vi "Set Dev Para wrapper.vi"(6 "iCurr":i32, 7 "iACR":i32, 8 "error in (no error)":errorcluster caption="错误输入（无错误）", 9 "iMCS":i32, 10 "dwCanNodeId":u32, 11 "dwDevIndex":u32) -> (0 "error out":errorcluster caption="错误输出", 3 "function return":u32)   [LabVIEW 2016, in "UISimCanFunc_wrapper.lvlib"]
doc: "_declspec (dllexport) DWORD SetDevPara_wrapper(DWORD dwDevIndex, DWORD dwCanNodeId, INT iMCS, INT iACR, INT iCurr);"
uses:
  <userlib>/UISimCanFunc_wrapper/UISimCanFunc_wrapper.lvlib
  <userlib>/UISimCanFunc_wrapper/UISimCanFunc_wrapper.dll
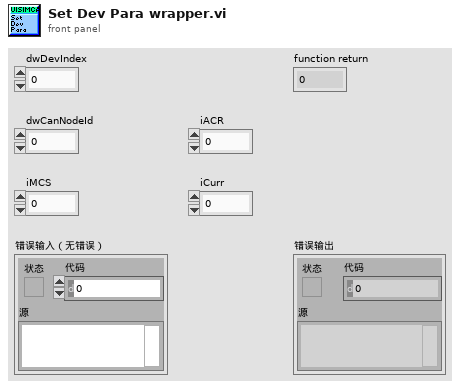
[diagram p1: front panel]
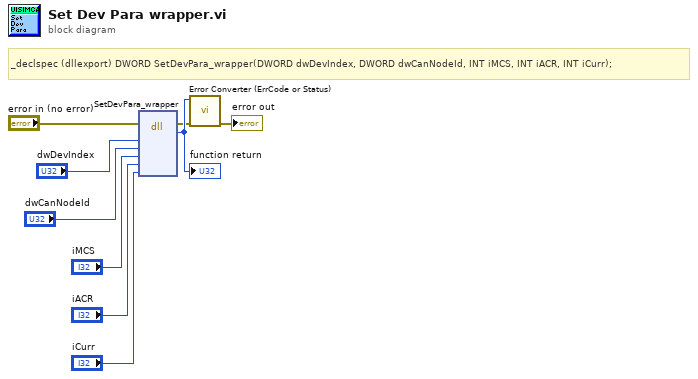
[diagram p0: block diagram]
diagram:
  # "_declspec (dllexport) DWORD SetDevPara_wrapper(DWORD dwDevIndex, DWORD dwCanNodeId, INT iMCS, INT iACR, INT iCurr);"
  n1 = dll-call lib="C:/Program Files (x86)/National Instruments/LabVIEW 2016/user.lib/UISimCanFunc_wrapper/UISimCanFunc_wrapper.*" fn="SetDevPara_wrapper"(error in="error in (no error)", "dwDevIndex"="dwDevIndex", "dwCanNodeId"="dwCanNodeId", "iMCS"="iMCS", "iACR"="iACR", "iCurr"="iCurr") -> (error out=w2:errorcluster, w9:u32)  [unwired: 7 in, 1 out]
  "function return" <- w9
  n2 = call <userlib>:"Error Converter (ErrCode or Status).vi"("error in (no error)"=w2, "error code"=w9) -> ("error out"=→"error out":errorcluster)  [unwired: 9 in]
